vi "Get Audio File Tags (Path).vi"(7 "Encoding (ASCII)":T1, 8 "error in (no error)":errorcluster, 11 "Path In":path) -> (0 "error out":errorcluster, 2 "Tags":string[](array[string]), 3 "Path Out":path)   [LabVIEW 2020, in "G-Audio.lvlib"]
doc: "Retrieve audio file tag data. Tags are returned as a string array, where each element is in the form FIELD=Value.\n\nNote that UTF-16 LE encoding is Windows only.\n\nSupported tag types:\nID3v2, ID3v1, Vorbis Comments, RIFF INFO"
uses:
  G-Audio.lvlib
  Controls/Text Encoding.ctl
  Private/Result To Error.vi
  <vilib>/Utility/error.llb/Error Cluster From Error Code.vi
  Unit Tests/UTF-8 To UTF-16.vi
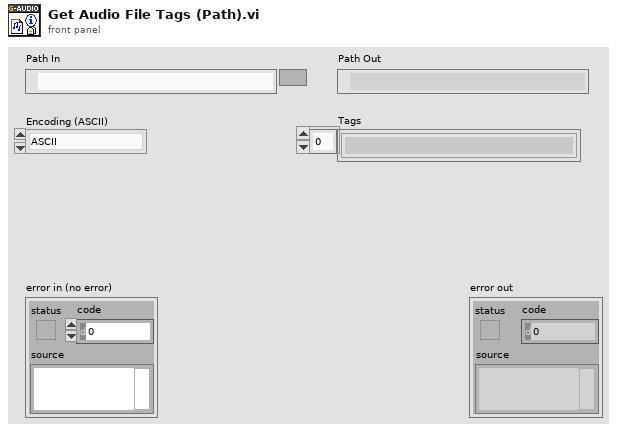
[diagram p1: front panel]
types:
  T1 = typedef "G-Audio.lvlib/Text Encoding.ctl" = enum16{"ASCII", "UTF-8", "UTF-16 LE"}
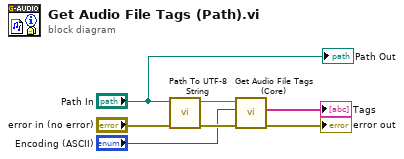
[diagram p0: block diagram]
diagram:
  n1 = call "Path To UTF-8 String.vi"("error in"="error in (no error)", "Path"="Path In") -> ("error out"=w3:errorcluster, "UTF-8 String"=w6:string)  [unwired: 8 in]
  n2 = call "Get Audio File Tags (Core).vi"("error in (no error)"=w3, "Encoding"="Encoding (ASCII)", "Path In"=w6) -> ("error out"=→"error out":errorcluster, "Tags"=→"Tags":string[])  [unwired: 6 in, 1 out]
  "Path Out" <- "Path In"
